vi "Signal_Pulse.vi"(1 "Input":bool) -> (0 "Output":bool)   [LabVIEW 2017]
doc: "Help by FRC Team 836 - The RoboBees\n\nThis VI is not finished. The output will always be false."
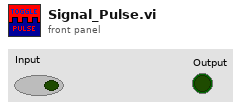
[diagram p1: front panel]
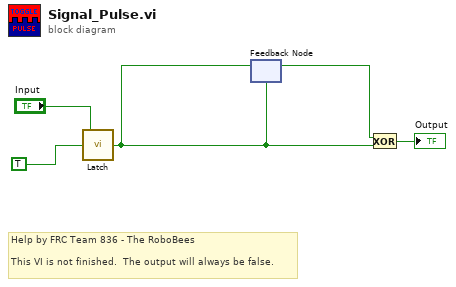
[diagram p0: block diagram]
diagram:
  # "Help by FRC Team 836 - The RoboBees\n\nThis VI is not finished.  The output will always be false."
  n1 = call <userlib>:"Latch.vi"("Edge"=TRUE, "In"="Input") -> ("Out"=w1:bool)
  n2 = feedback-in #1(w1) -> ()
  n3 = feedback #1(w1) -> (w2:bool)
  n4 = Exclusive Or(1:w1, 2:w2) -> (0:→"Output":bool)
